vi "Get SCL Selected Item.vi"(8 "error in":errorcluster, 11 "SCL":refnum<vi>) -> (0 "error out":errorcluster, 2 "Selected Item (Index)":i32, 3 "Selected Item (String)":string)   [LabVIEW 2021]
doc: "Gets the item that is currently selected in an SCL.\n\nSCL = Single-Column Listbox"
panel:
  # "Development\ncontrols/indicators useful for development and testing, but which are not outputs of the VI"
  # "Input\nInputs to the VI"
  # "Output\nOutputs of the VI"
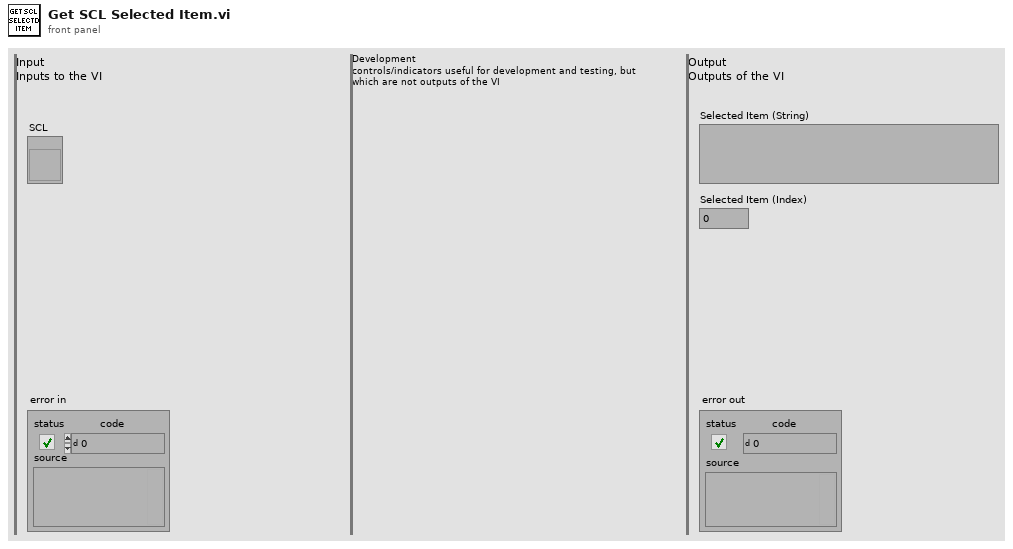
[diagram p1: front panel]
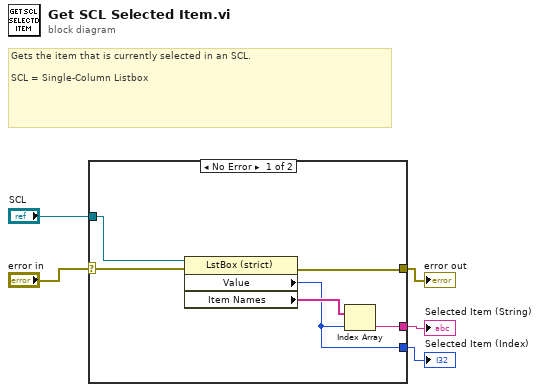
[diagram p0: block diagram]
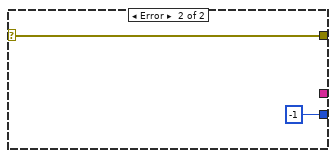
[diagram p2: hidden frame]
diagram:
  # "Gets the item that is currently selected in an SCL.\n\nSCL = Single-Column Listbox"
  n1 = case shown="No Error" "error in" {
    selector: "error in" -> [w11 w13]
    tunnel: [w9 w13] -> w4
    tunnel: "SCL" -> [w10 _]
    tunnel: [w7 _] -> w2
    tunnel: [w6 -1 ("Value")] -> w1
    frame No Error {
      n2 = property class="LstBox (strict)"(reference=w10, error in=w11) -> (error out=w9:errorcluster, "Value"=w6:i32, "Item Names"=w8:string[])  [unwired: 1 out]
      n3 = Index Array(array=w8, index=w6) -> (element=w7:string)
    }
    frame Error {
    }
  }
  "error out" <- w4
  "Selected Item (String)" <- w2
  "Selected Item (Index)" <- w1
